vi "Load.vi"   [LabVIEW 2020, in "NI_XML.lvlib"]
doc: "Opens an XML file and allows you to configure the XML parser to validate the file against a schema or Document Type Definition (DTD).\n\nNational Instruments recommends that you use the Close VI to close all the references after using the XML parser classes."
uses:
  <vilib>/xml/NI_XML.lvlib
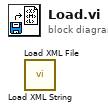
[diagram p0: block diagram]
diagram:
  n1 = call <vilib>:"Load XML String.vi"() -> ()  [unwired: 13 in, 3 out]
  n2 = call <vilib>:"Load XML File.vi"() -> ()  [unwired: 13 in, 3 out]
